vi "Configure RT FIFO Write.vi"(8 "error in (no error)":errorcluster, 10 "Ouput Values Array":dbl[](array[numeric]), 11 "Device Ref in":T1 format="%.0x") -> (0 "error out":errorcluster, 2 "RT FIFO Write out":refnum<k33>, 3 "Device Ref out":T1 format="%.0x")   [LabVIEW 2012, in "Shared Variable Custom Device.lvlib"]
uses:
  Shared Variable Custom Device.lvlib
  <vilib>/NI Veristand/Custom Device API/Custom Device Item Ref.ctl
  <vilib>/NI Veristand/Custom Device API/Custom Device API.lvlib
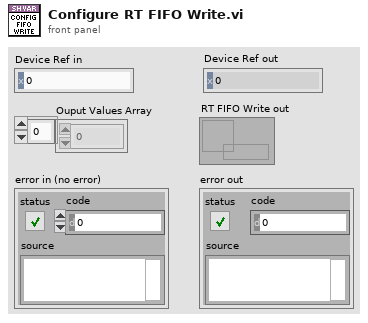
[diagram p1: front panel]
types:
  T1 = typedef "Custom Device API.lvlib/Custom Device Item Ref.ctl" = u64
  T2 = cluster{"read mode":enum16{"polling", "blocking"}, "write mode":enum16{"polling", "blocking"}}
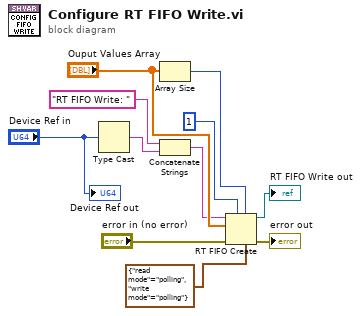
[diagram p0: block diagram]
diagram:
  n1 = Type Cast(x="Device Ref in") -> (*(type *) &x=w1:string)  [unwired: 1 in]
  n2 = Array Size(array="Ouput Values Array") -> (size(s)=w5:i32)
  n3 = Concatenate Strings("RT FIFO Write: " ("string"), w1) -> (w4:string)
  n4 = RT FIFO Create(0:w4, 1:"Ouput Values Array", 3:"error in (no error)", 4:u32 1 ("size (10)"), 6:w5, 7:T2 {"read mode"=enum."polling", "write mode"=enum."polling"} ("r/w modes (polling,polling)")) -> (8:→"RT FIFO Write out":refnum<k33>, 11:→"error out":errorcluster)  [unwired: 2 in, 1 out]
  "Device Ref out" <- "Device Ref in"
